vi "生成CODMn data (子VI).vi"() -> (3 "data":T1)   [LabVIEW 2016, in "斯坦道CODMn.lvlib"]
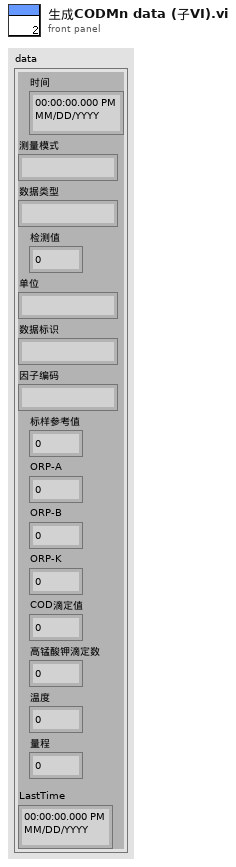
[diagram p1: front panel]
types:
  T1 = cluster{"时间":timestamp, "测量模式":string, "数据类型":string, "检测值":sgl, "单位":string, "数据标识":string, "因子编码":string, "标样参考值":sgl, "ORP-A":sgl, "ORP-B":sgl, "ORP-K":sgl, "COD滴定值":sgl, "高锰酸钾滴定数":sgl, "温度":sgl, "量程":sgl, "LastTime":timestamp}
  T2 = cluster{"运行模式":enum16{"维护模式", "常规模式", "应急模式", "质控模式"}}
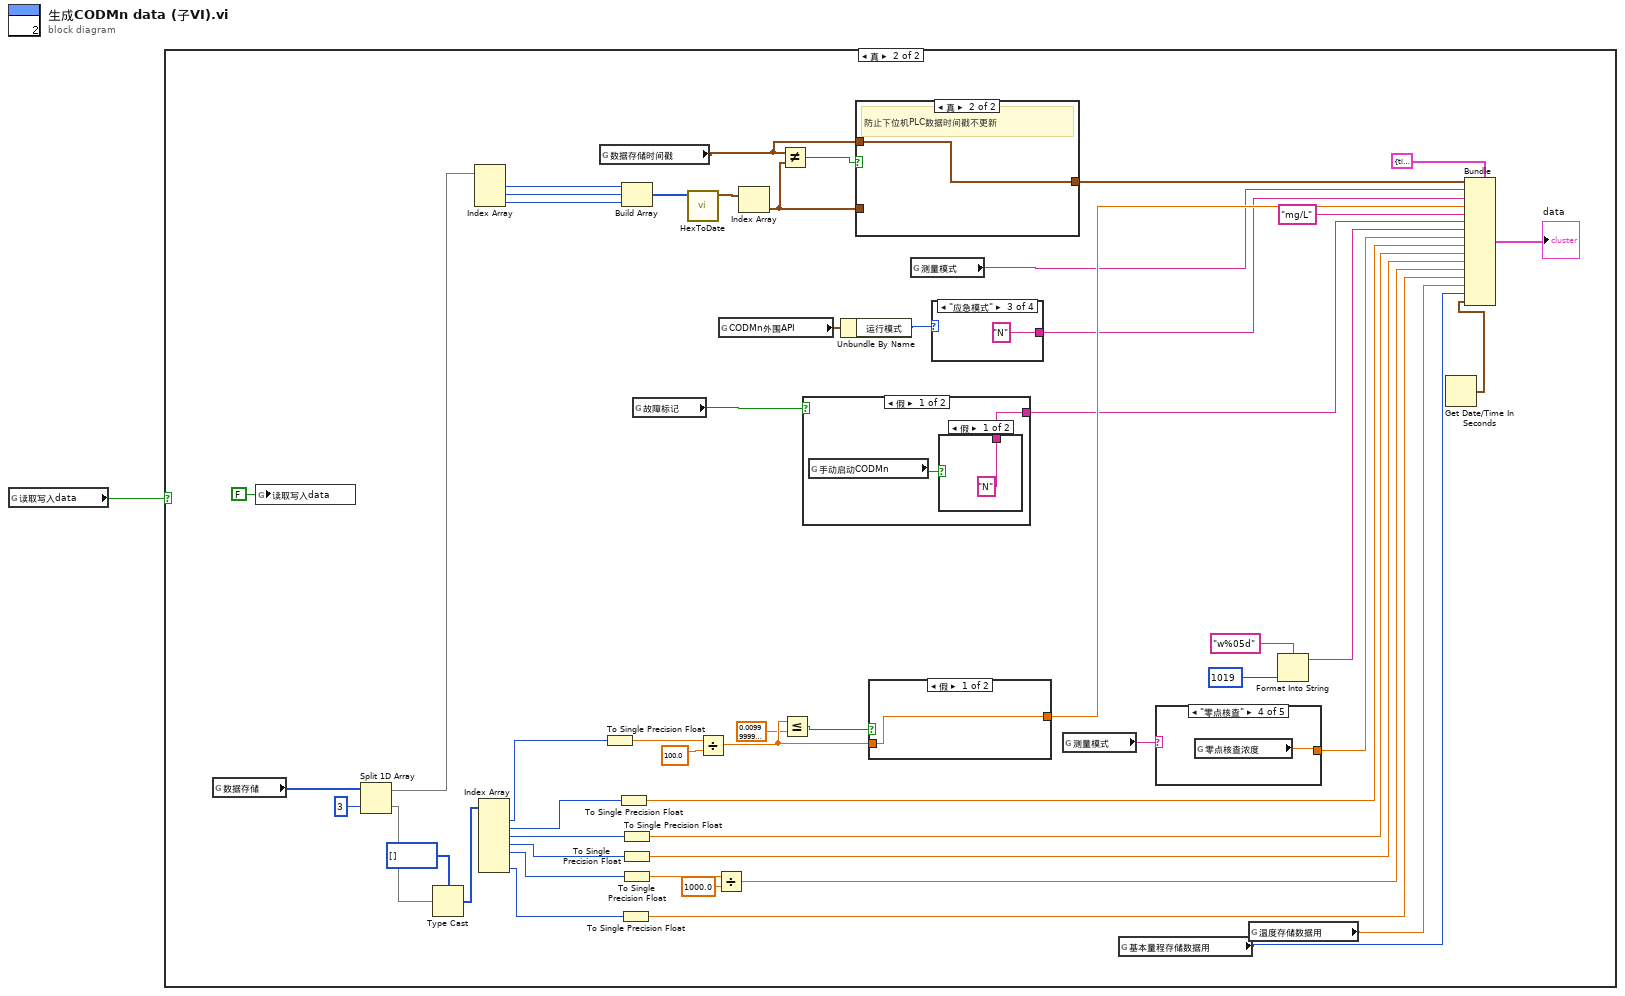
[diagram p0: block diagram]
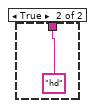
[diagram p4: hidden frame]
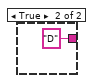
[diagram p5: hidden frame]
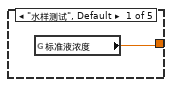
[diagram p6: hidden frame]
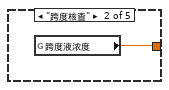
[diagram p7: hidden frame]
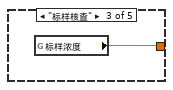
[diagram p8: hidden frame]
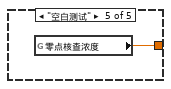
[diagram p9: hidden frame]
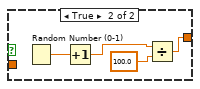
[diagram p10: hidden frame]
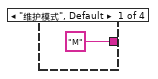
[diagram p11: hidden frame]
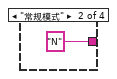
[diagram p12: hidden frame]
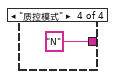
[diagram p13: hidden frame]
diagram:
  n1 = global read "COD读取DATA全局.vi" "读取写入data"() -> (w1:bool)
  n2 = case shown="真" w1 {
    frame False {
    }
    frame True {
      n3 = global read "COD读取DATA全局.vi" "数据存储"() -> (w4:u16[])
      n4 = global write "COD读取DATA全局.vi" "读取写入data"(FALSE ("读取写入data")) -> ()
      n5 = Split 1D Array(array=w4, index=3 ("索引")) -> (first subarray=w12:u16[], second subarray=w3:u16[])
      n6 = Type Cast(type=i16[] [], x=w3) -> (*(type *) &x=w2:i16[])
      n7 = Index Array(array=w12) -> (element #1=w14:u16, element #2=w15:u16, element #3=w16:u16)  [unwired: 3 in]
      n8 = Index Array(array=w2) -> (element #1=w40:i16, element #2=w18:i16, element #3=w19:i16, element #4=w20:i16, element #5=w21:i16, element #7=w50:i16)  [unwired: 7 in, 1 out]
      n9 = global read "COD读取DATA全局.vi" "数据存储时间戳"() -> (w51:timestamp)
      n10 = To Single Precision Float(number=w40) -> (single precision float=w38:sgl)
      n11 = To Single Precision Float(number=w18) -> (single precision float=w30:sgl)
      n12 = To Single Precision Float(number=w50) -> (single precision float=w35:sgl)
      n13 = Build Array(w14, w15, w16) -> (w17:u16[])
      n14 = To Single Precision Float(number=w19) -> (single precision float=w29:sgl)
      n15 = To Single Precision Float(number=w20) -> (single precision float=w28:sgl)
      n16 = To Single Precision Float(number=w21) -> (single precision float=w24:sgl)
      n17 = global read "COD读取DATA全局.vi" "故障标记"() -> (w53:bool)
      n18 = call "HexToDate.vi"("数组"=w17) -> ("DATE"=w13:timestamp[])  [unwired: 10 in]
      n19 = Divide(x=w38, y=sgl 100.0) -> (x/y=w39:sgl)
      n20 = Divide(x=w24, y=sgl 1000.0) -> (x/y=w27:sgl)
      n21 = global read "CODMN外部API.vi" "CODMn外围API"() -> (w43:T2)
      n22 = Index Array(array=w13) -> (element=w46:timestamp)  [unwired: 1 in]
      n23 = Not Equal?(x=w51, y=w46) -> (x != y?=w47:bool)
      n24 = Less Or Equal?(x=w39, y=sgl 0.01) -> (x <= y?=w37:bool)
      n25 = case shown="假" w53 {
        tunnel: [w57 "D" ("数据标识")] -> w32
        frame False {
          n26 = global read "CODMN外部API.vi" "手动启动CODMn"() -> (w56:bool)
          n27 = case shown="假" w56 {
            tunnel: ["N" ("数据标识") "hd" ("数据标识")] -> w57
            frame False {
            }
            frame True {
            }
          }
        }
        frame True {
        }
      }
      n28 = Unbundle By Name(w43) -> ("运行模式"=w44:enum16{"维护模式", "常规模式", "应急模式", "质控模式"})
      n29 = case "条件结构" shown="真" w47 {
        tunnel: w46 -> [w54 _]
        tunnel: w51 -> [_ w55]
        tunnel: [w54 w55] -> w48
        frame False {
        }
        frame True {
          # "防止下位机PLC数据时间戳不更新"
        }
      }
      n30 = case shown="假" w37 {
        tunnel: [w66 w67] -> w49
        tunnel: w39 -> [w66 _]
        frame False {
        }
        frame True {
          n31 = Random Number (0-1)() -> (number: 0 to 1=w70:dbl)
          n32 = Increment(x=w70) -> (x+1=w68:dbl)
          n33 = Divide(x=w68, y=sgl 100.0) -> (x/y=w67:dbl)
        }
      }
      n34 = global read "COD测量模式全局.vi" "测量模式"() -> (w45:string)
      n35 = case shown="\"应急模式\"" w44 {
        tunnel: ["M" ("单位") "N" ("单位") "N" ("单位") "N" ("单位")] -> w34
        frame "维护模式", Default {
        }
        frame "常规模式" {
        }
        frame "应急模式" {
        }
        frame "质控模式" {
        }
      }
      n36 = global read "COD测量模式全局.vi" "测量模式"() -> (w41:string)
      n37 = global read "COD读取DATA全局.vi" "基本量程存储数据用"() -> (w10:enum16{"L", "H"})
      n38 = case shown="\"零点核查\"" w41 {
        tunnel: [w61 w62 w63 w64 w65] -> w42
        frame "水样测试", Default {
          n39 = global read "COD浓度全局变量.vi" "标准液浓度"() -> (w61:dbl)
        }
        frame "跨度核查" {
          n40 = global read "CODMn断电保存全局变量.vi" "跨度液浓度"() -> (w62:dbl)
        }
        frame "标样核查" {
          n41 = global read "CODMn断电保存全局变量.vi" "标样浓度"() -> (w63:dbl)
        }
        frame "零点核查" {
          n42 = global read "CODMn断电保存全局变量.vi" "零点核查浓度"() -> (w64:dbl)
        }
        frame "空白测试" {
          n43 = global read "CODMn断电保存全局变量.vi" "零点核查浓度"() -> (w65:dbl)
        }
      }
      n44 = global read "COD读取DATA全局.vi" "温度存储数据用"() -> (w52:dbl)
      n45 = Format Into String(format string="w%05d" ("格式字符串"), u32 1019 ("因子编码")) -> (resulting string=w31:string)  [unwired: 2 in, 1 out]
      n46 = Get Date/Time In Seconds() -> (seconds since 1Jan1904=w6:timestamp)
      n47 = Bundle(cluster=T1 {"时间"=timestamp(0 s since 1904-01-01), "测量模式"="", "数据类型"="", "检测值"=0.0, "单位"="", "数据标识"="", "因子编码"="", "标样参考值"=0.0, "ORP-A"=0.0, "ORP-B"=0.0, "ORP-K"=0.0, "COD滴定值"=0.0, "高锰酸钾滴定数"=0.0, "温度"=0.0, "量程"=0.0, "LastTime"=timestamp(0 s since 1904-01-01)} ("data"), "时间"=w48, "测量模式"=w45, "数据类型"=w34, "检测值"=w49, "单位"="mg/L", "数据标识"=w32, "因子编码"=w31, "标样参考值"=w42, "ORP-A"=w30, "ORP-B"=w29, "ORP-K"=w28, "COD滴定值"=w27, "高锰酸钾滴定数"=w35, "温度"=w52, "量程"=w10, "LastTime"=w6) -> (→"data":T1)
    }
  }
